vi "input.vi"(8 "error in":errorcluster, 10 "data table in":T1, 11 "Tag Bus Web Interface runtime in":refnum<class "Tag Bus Web Interface runtime.lvclass">) -> (0 "error out":errorcluster, 2 "data table out":T1, 3 "Tag Bus Web Interface runtime out":refnum<class "Tag Bus Web Interface runtime.lvclass">)   [LabVIEW 2013, in "Tag Bus Web Interface runtime.lvclass"]
doc: "Provides an interface for reading data from a module at runtime. While this interface performs no operations, a child should provide an override which may read from any open sessions, references, or interfaces."
uses:
  Tag Bus Web Interface runtime.lvclass
  <vilib>/NI/Tag Bus/table/data table.ctl
  Tag Bus Web Interface runtime.lvclass/Tag Bus Web Interface runtime.ctl
  <vilib>/NI/Tag Bus/table/data table.lvlib
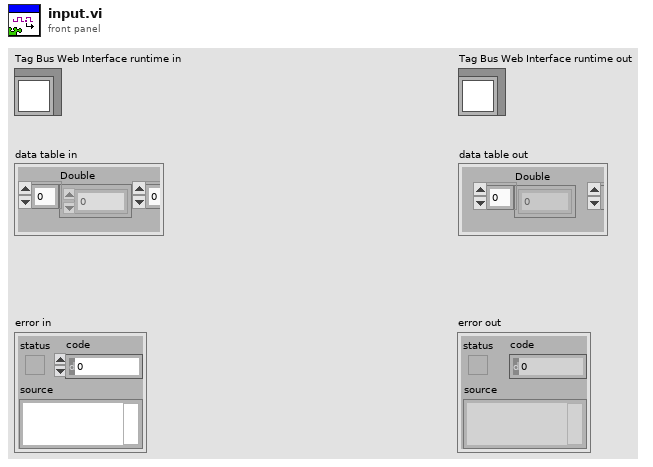
[diagram p1: front panel]
types:
  T1 = typedef "tag bus.lvlib/data table.lvlib/data table.ctl" = cluster{"Double":dbl[], "Single":sgl[], "I64":i64[], "I32":i32[], "I16":i16[], "I8":i8[], "U64":u64[], "U32":u32[], "U16":u16[], "U8":u8[], "Boolean":bool[], "String":string[], "Array of Double":cluster{"DBL Array":dbl[]}[], "Array of Single":cluster{"SGL Array":sgl[]}[], "Array of I64":cluster{"I64 Array":i64[]}[], "Array of I32":cluster{"I32 Array":i32[]}[], "Array of I16":cluster{"I16 Array":i16[]}[], "Array of I8":cluster{"I8 Array":i8[]}[], "Array of U64":cluster{"U64 Array":u64[]}[], "Array of U32":cluster{"U32 Array":u32[]}[], "Array of U16":cluster{"U16 Array":u16[]}[], "Array of U8":cluster{"U8 Array":u8[]}[], "Array of Boolean":cluster{"Boolean Array":bool[]}[], "Array of String":cluster{"String Array":string[]}[]}
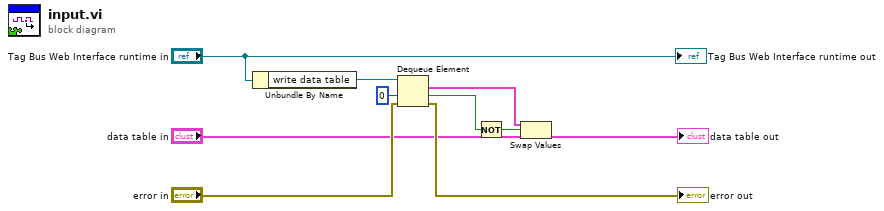
[diagram p0: block diagram]
diagram:
  n1 = Unbundle By Name("Tag Bus Web Interface runtime in") -> ("write data table"=w9:refnum<queue>)
  n2 = Dequeue Element(queue=w9, timeout in ms (-1)=0, error in (no error)="error in") -> (element=w4:T1, timed out?=w2:bool, error out=→"error out":errorcluster)  [unwired: 1 out]
  n3 = Not(x=w2) -> (.not. x?=w3:bool)
  n4 = Swap Values(12:w4, 13:w3, 14:"data table in") -> (3:→"data table out":T1)  [unwired: 1 out]
  "Tag Bus Web Interface runtime out" <- "Tag Bus Web Interface runtime in"
